vi "Add Scaling.vi"(1 "Digitizer 2 Waveforms":T1(array[cluster]), 2 "Digitizer 1 Waveforms":T1(array[cluster]), 3 "Add Tegam Scaling?":bool, 4 "Digitizer 1 Gain Multiplier":dbl=nan) -> (0 "Waveforms Out":T1(array[cluster]))   [LabVIEW 2010]
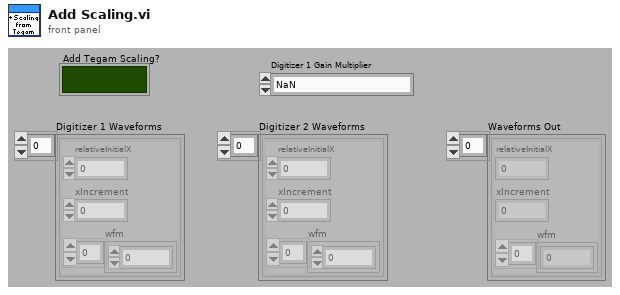
[diagram p1: front panel]
types:
  T1 = cluster{"relativeInitialX":dbl, "xIncrement":dbl, "wfm":dbl[]}[]
  T2 = cluster{"relativeInitialX":dbl, "xIncrement":dbl, "wfm":dbl[]}
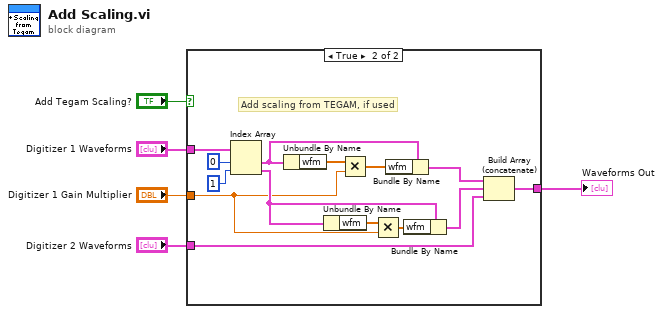
[diagram p0: block diagram]
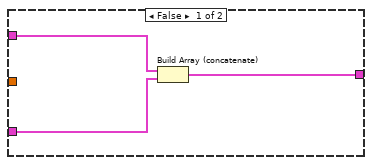
[diagram p2: hidden frame]
diagram:
  n1 = case shown="True" "Add Tegam Scaling?" {
    tunnel: "Digitizer 1 Waveforms" -> [w8 w22]
    tunnel: "Digitizer 1 Gain Multiplier" -> [_ w10]
    tunnel: "Digitizer 2 Waveforms" -> [w7 w15]
    tunnel: [w6 w14] -> w4
    frame False {
      n2 = Build Array (concatenate)(w8, w7) -> (w6:T1)
    }
    frame True {
      # "Add scaling from TEGAM, if used"
      n3 = Index Array(array=w22, index #1=0 ("index"), index #2=1 ("index")) -> (element #1=w19:T2, element #2=w11:T2)
      n4 = Unbundle By Name(w19) -> ("wfm"=w21:dbl[])
      n5 = Unbundle By Name(w11) -> ("wfm"=w12:dbl[])
      n6 = Multiply(x=w21, y=w10) -> (x*y=w18:dbl[])
      n7 = Multiply(x=w12, y=w10) -> (x*y=w13:dbl[])
      n8 = Bundle By Name(cluster=w19, "wfm"=w18) -> (w16:T2)
      n9 = Bundle By Name(cluster=w11, "wfm"=w13) -> (w9:T2)
      n10 = Build Array (concatenate)(w16, w9, w15) -> (w14:T1)
    }
  }
  "Waveforms Out" <- w4
